vi "even_number_Property_node.vi"() -> ()   [LabVIEW 2019]
panel:
  in  "stop":bool
  in  "Numeric":dbl
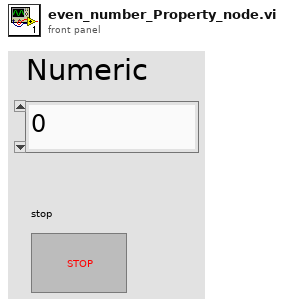
[diagram p1: front panel]
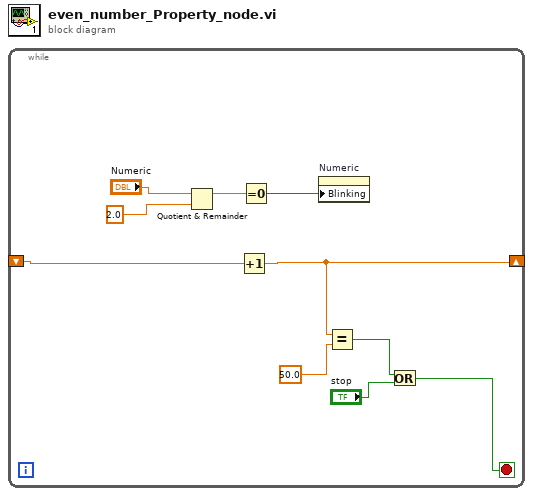
[diagram p0: block diagram]
diagram:
  n1 = while {
    shift-right: [w4] -> _
    shift-left: _ -> [w6]
    stop <- w1 stop-if-true
    n2 = Quotient & Remainder(x="Numeric", y=2.0) -> (x-y*floor(x/y)=w7:dbl)  [unwired: 1 out]
    n3 = Increment(x=w6) -> (x+1=w4:dbl)
    n4 = Equal To 0?(x=w7) -> (x = 0?=w10:bool)
    n5 = property on="Numeric" class="DigNum (strict)"("Blinking"=w10) -> ()  [unwired: 2 in, 2 out]
    n6 = Equal?(x=w4, y=50.0) -> (x = y?=w3:bool)
    n7 = Or(x=w3, y="stop") -> (x .or. y?=w1:bool)
  }
